vi "Check Status.vi"(8 "error in (no error)":errorcluster, 11 "Fluke Calibrator in":refnum<class "Fluke Calibrator.lvclass">) -> (0 "error out":errorcluster, 1 "Status":string, 2 "Ready?":bool, 3 "Fluke Calibrator out":refnum<class "Fluke Calibrator.lvclass">)   [LabVIEW 2012, in "Fluke Calibrator.lvclass"]
doc: "(Dynamic) Check if the instrument is powered on and update its member fields with the instrument's current status. Optionally return a text status message."
uses:
  Fluke Calibrator.lvclass
  Utility Classes/Readable/Readable.lvclass
panel:
  out "Output":bool
  out "Voltage":dbl format="%_6g"
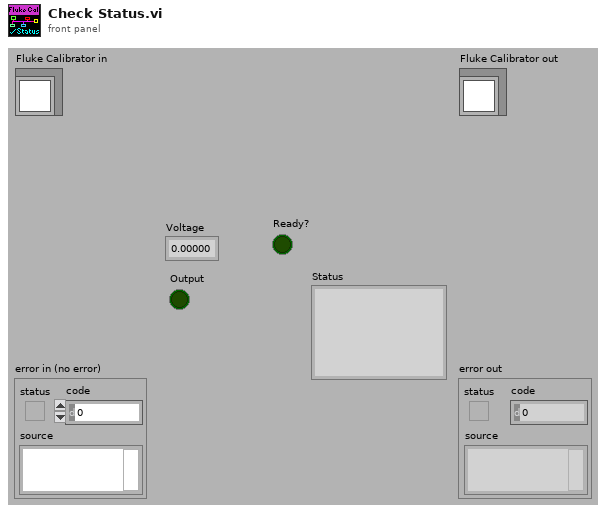
[diagram p1: front panel]
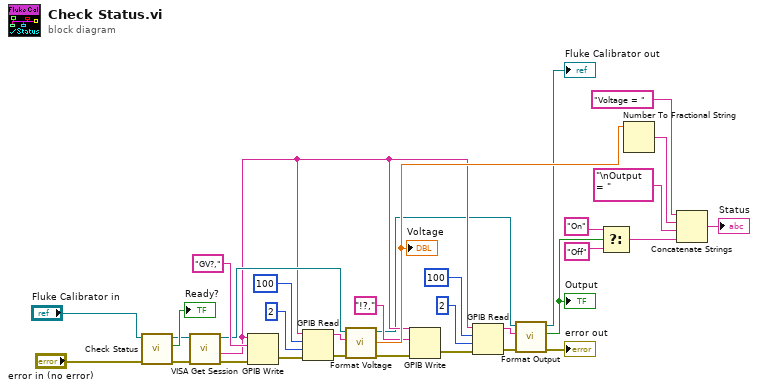
[diagram p0: block diagram]
diagram:
  n1 = call-parent "Check Status.vi"("error in (no error)"="error in (no error)", "Instrument in"="Fluke Calibrator in") -> ("error out"=w29:errorcluster, "Ready?"=→"Ready?":bool, "Instrument out"=w30:refnum<class "Fluke Calibrator.lvclass">)  [unwired: 6 in, 1 out]
  n2 = call-dynamic "VISA Get Session.vi"("error in (no error)"=w29, "Instrument.lvclass in"=w30) -> ("error out"=w28:errorcluster, "GPIB string"=w11:string, "Instrument.lvclass out"=w21:refnum<class "Fluke Calibrator.lvclass">)  [unwired: 6 in, 1 out]
  n3 = GPIB Write(0:w11, 1:"GV?," ("write buffer"), 3:w28) -> (6:w24:errorcluster)  [unwired: 2 in, 1 out]
  n4 = GPIB Read(0:w11, 1:100 ("byte count"), 2:i16 2 ("mode (0)"), 3:w24) -> (5:w22:string, 7:w23:errorcluster)  [unwired: 1 in, 1 out]
  n5 = call "Format Voltage.vi"("error in (no error)"=w23, "String In"=w22, "Fluke Calibrator in"=w21) -> ("error out"=w12:errorcluster, "Number out"=w20:dbl, "Fluke Calibrator out"=w7:refnum<class "Fluke Calibrator.lvclass">)  [unwired: 6 in]
  "Voltage" <- w20
  n6 = GPIB Write(0:w11, 1:"!?," ("data"), 3:w12) -> (6:w15:errorcluster)  [unwired: 2 in, 1 out]
  n7 = GPIB Read(0:w11, 1:100 ("byte count"), 2:i16 2 ("mode (0)"), 3:w15) -> (5:w6:string, 7:w5:errorcluster)  [unwired: 1 in, 1 out]
  n8 = call "Format Output.vi"("error in (no error)"=w5, "Input"=w6, "Fluke Calibrator in"=w7) -> ("error out"=→"error out":errorcluster, "Output"=w1:bool, "Fluke Calibrator out"=→"Fluke Calibrator out":refnum<class "Fluke Calibrator.lvclass">)  [unwired: 6 in]
  "Output" <- w1
  n9 = Select(t="On", s=w1, f="Off") -> (s? t:f=w2:string)
  n10 = Number To Fractional String(number=w20) -> (F-format string=w17:string)  [unwired: 3 in]
  n11 = Concatenate Strings("Voltage = ", w17, "\nOutput = ", w2) -> (→"Status":string)
